vi "Ctor.vi"(8 "error in (no error)":errorcluster) -> (0 "error out":errorcluster, 3 "App out":refnum<class "App.lvclass">)   [LabVIEW 2020, in "App.lvclass"]
uses:
  App.lvclass
  Blueprint Qty.ctl
  Blueprint/Blueprint.lvclass
  App.lvclass/App.ctl
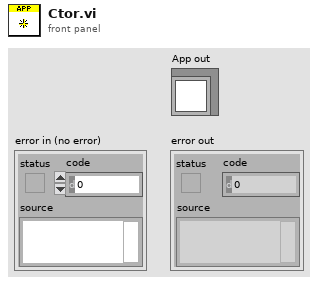
[diagram p1: front panel]
types:
  T1 = typedef "App.lvclass/Blueprint Qty.ctl" = cluster{"Blueprint":refnum<class "Blueprint.lvclass">, "Qty":dbl}
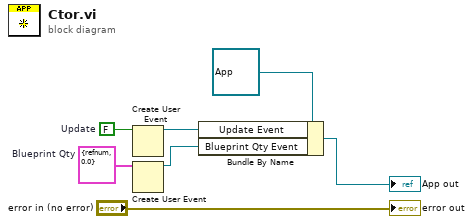
[diagram p0: block diagram]
diagram:
  w2 = T1 {"Blueprint"=refnum, "Qty"=0.0}  # Blueprint Qty
  w4 = FALSE  # Update
  n1 = Create User Event(user event datatype=w4) -> (user event=w3:refnum<user-event>)  [unwired: 1 in, 1 out]
  n2 = Create User Event(user event datatype=w2) -> (user event=w1:refnum<user-event>)  [unwired: 1 in, 1 out]
  n3 = Bundle By Name(cluster=refnum<class "App.lvclass"> refnum ("App in"), "Update Event"=w3, "Blueprint Qty Event"=w1) -> (→"App out":refnum<class "App.lvclass">)
  "error out" <- "error in (no error)"
